vi "FGV_LoopCSV.vi"(8 "error in (no error)":errorcluster, 9 "Cluster":T1={"IncioPrograma"=FALSE, "Estado"=enum."Start", "Com_Escribir"=enum."GET REF", "array25_tramas"=[]}, 10 "CSV_State_In":T2=enum."Idle", 11 "FGV_Action":T9) -> (0 "error out":errorcluster, 1 "Cluster 2":T1={"IncioPrograma"=FALSE, "Estado"=enum."Start", "Com_Escribir"=enum."GET REF", "array25_tramas"=[]}, 2 "CSV_State_Out":T2=enum."Idle")   [LabVIEW 2026]
uses:
  Ctrl_Estados.ctl
  Control/Ctrl_Errores.ctl
  Control/Ctrl_Motores_Valores.ctl
  Control/Ctrl_datos6motores_final.ctl
  Control/Ctr_Enc_Values.ctl
  Control/Ctrl_Array_Enc_Out_final.ctl
  Control/Ctrl_EscrituraComandos.ctl
  Control/Ctrl_DataLoggerQueue.ctl
  Ctrl_CSVLoop.ctl
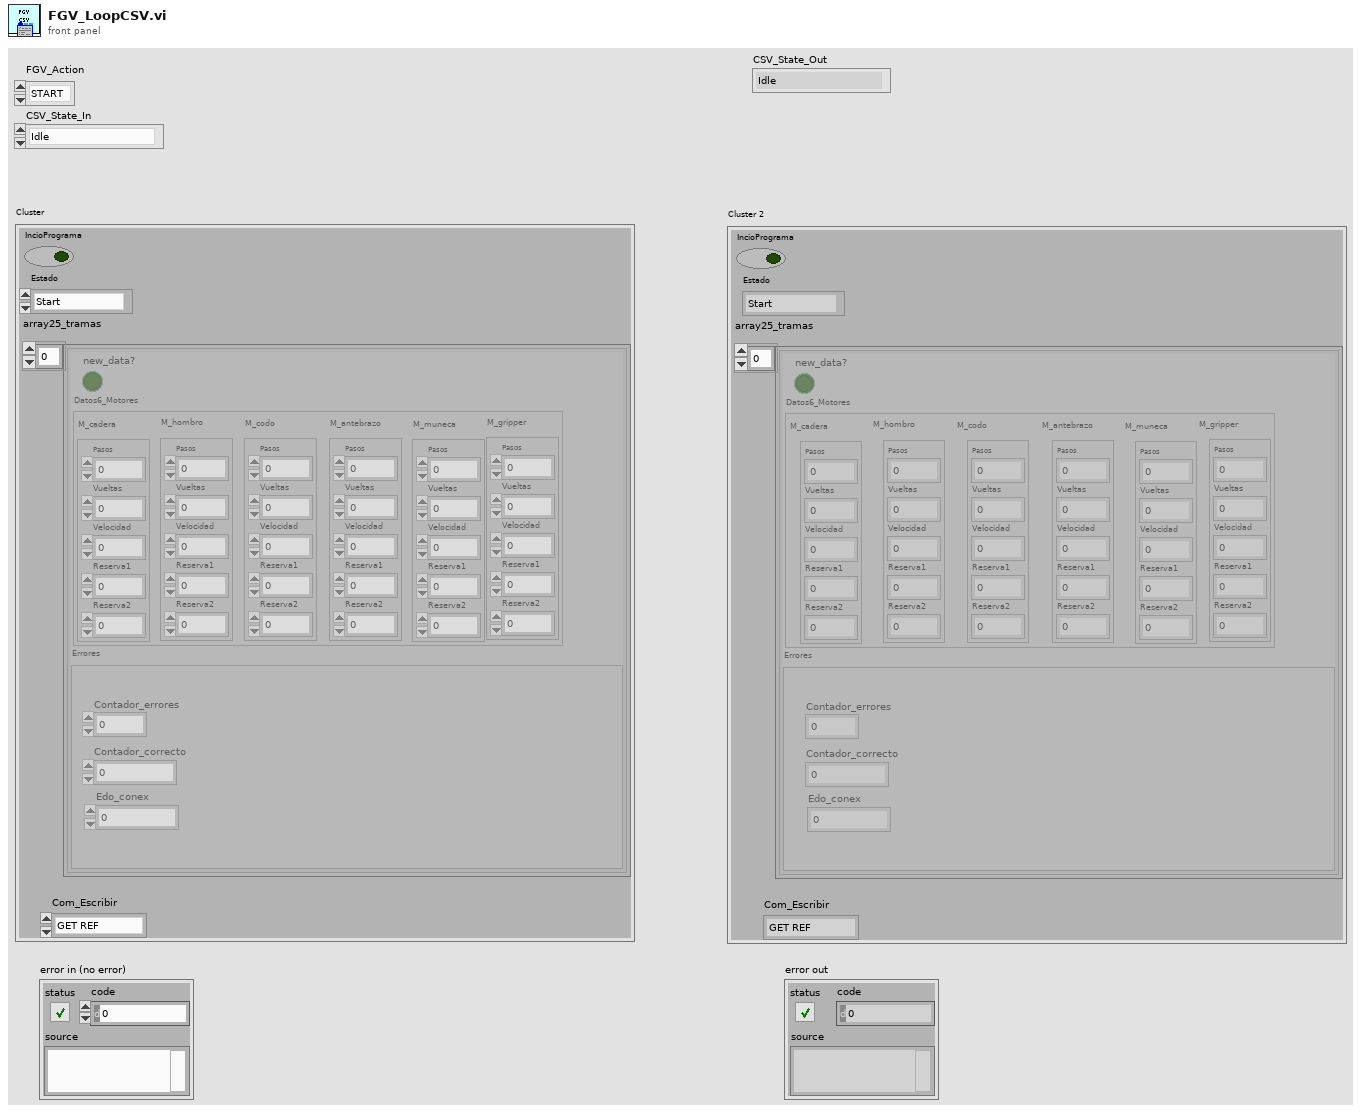
[diagram p1: front panel]
types:
  T1 = typedef "Ctrl_DataLoggerQueue.ctl" = cluster{"IncioPrograma":bool, "Estado":T2, "Com_Escribir":T3, "array25_tramas":T4}
  T2 = typedef "Ctrl_Estados.ctl" = enum16{"Show_Control", "LogData", "Idle", "SHOW PID", "PID_GUI", "Stop", "Show_Dashboard", "Reconnect", "Log_Data_All", "Start", "WRITE_DATA", "SEND_COM"}
  T3 = typedef "Ctrl_EscrituraComandos.ctl" = enum16{"GET REF", "SEND ROUTINE", "MOVE MANUAL", "SEND ESP32", "SET REF"}
  T4 = typedef "Ctrl_Array_Enc_Out_final.ctl" = T5[]
  T5 = typedef "Ctr_Enc_Values.ctl" = cluster{"Datos6_Motores":T6, "Errores":T8, "new_data?":bool}
  T6 = typedef "Ctrl_datos6motores_final.ctl" = cluster{"M_cadera":T7, "M_hombro":T7, "M_codo":T7, "M_antebrazo":T7, "M_muneca":T7, "M_gripper":T7}
  T7 = typedef "Ctrl_Motores_Valores.ctl" = cluster{"Pasos":i32, "Vueltas":i16, "Velocidad":dbl, "Reserva1":u8, "Reserva2":u8}
  T8 = typedef "Ctrl_Errores.ctl" = cluster{"Contador_correcto":u32, "Contador_errores":u32, "Edo_conex":u32}
  T9 = typedef "Ctrl_CSVLoop.ctl" = enum16{"START", "SET DATA", "STOP", "SET STATE", "GET STATE"}
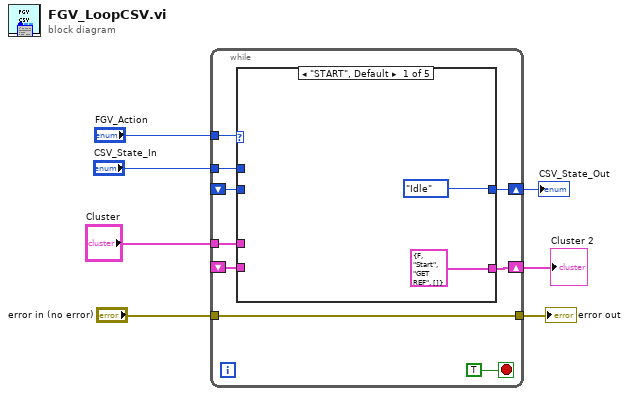
[diagram p0: block diagram]
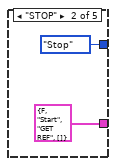
[diagram p2: hidden frame]
diagram:
  n1 = while {
    tunnel: "error in (no error)" -> [w15]
    tunnel: [w15] -> w6
    tunnel: "FGV_Action" -> [w14]
    shift-right: [w13] -> w4
    shift-left: _ -> [w11]
    tunnel: "CSV_State_In" -> [w12]
    tunnel: "Cluster" -> [w10]
    shift-right: [w9] -> w1
    shift-left: _ -> [w8]
    stop <- TRUE stop-if-true
    n2 = case shown="\"START\", Default" w14 {
      tunnel: [Ctrl_Estados."Idle" ("CSV_State_In") Ctrl_Estados."Stop" ("CSV_State_In") w22 w23 w26] -> w13
      tunnel: w12 -> [_ _ w22 _ _]
      tunnel: w11 -> [_ _ _ w23 w26]
      tunnel: w10 -> [_ _ _ w24 _]
      tunnel: [T1 {"IncioPrograma"=FALSE, "Estado"=enum."Start", "Com_Escribir"=enum."GET REF", "array25_tramas"=[]} ("Cluster") T1 {"IncioPrograma"=FALSE, "Estado"=enum."Start", "Com_Escribir"=enum."GET REF", "array25_tramas"=[]} ("Cluster") w21 w24 w25] -> w9
      tunnel: w8 -> [_ _ w21 _ w25]
      frame "START", Default {
      }
      frame "STOP" {
      }
      frame "SET STATE" {
      }
      frame "SET DATA" {
      }
      frame "GET STATE" {
      }
    }
  }
  "error out" <- w6
  "CSV_State_Out" <- w4
  "Cluster 2" <- w1
